vi "1.vi"() -> ()   [LabVIEW 2016]
panel:
  in  "B1 2":bool
  in  "espera 2":u32
  out "indice 2":i32
  out "Waveform Chart 2":dbl(graph)
  out "Waveform Chart":dbl(graph)
  out "indice 1":i32
  in  "espera 1":u32
  in  "B1":bool
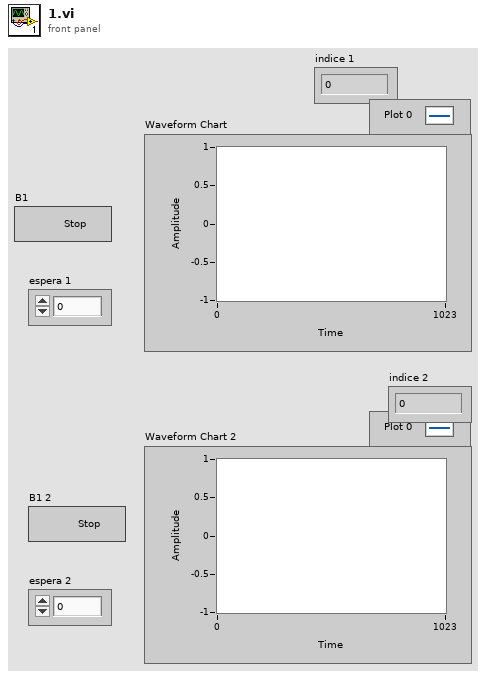
[diagram p1: front panel]
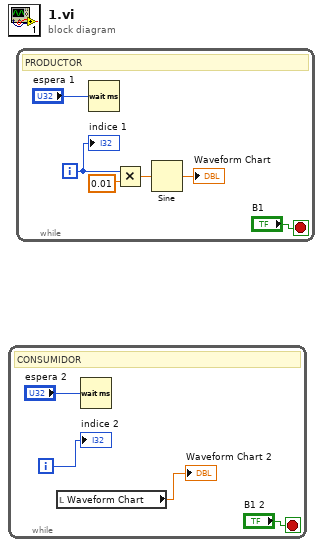
[diagram p0: block diagram]
diagram:
  n1 = while {
    i -> [w2]
    stop <- "B1 2" stop-if-true
    # "CONSUMIDOR"
    n2 = local read "Waveform Chart"() -> (→"Waveform Chart 2":dbl)
    n3 = Wait (ms)(milliseconds to wait="espera 2") -> ()  [unwired: 1 out]
    "indice 2" <- w2
  }
  n4 = while {
    i -> [w8]
    stop <- "B1" stop-if-true
    # "PRODUCTOR"
    n5 = Wait (ms)(milliseconds to wait="espera 1") -> ()  [unwired: 1 out]
    n6 = Multiply(x=w8, y=0.01) -> (x*y=w7:dbl)
    n7 = Sine(x=w7) -> (sin(x)=→"Waveform Chart":dbl)
    "indice 1" <- w8
  }
